vi "Calculate Derived Data.vi"(8 "error in":errorcluster, 11 "CVT":map{string, string}(c390)) -> (0 "error out":errorcluster, 3 "CVT Out":map{string, dbl}(c390))   [LabVIEW 2025]
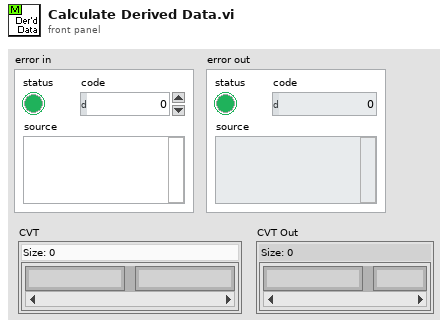
[diagram p1: front panel]
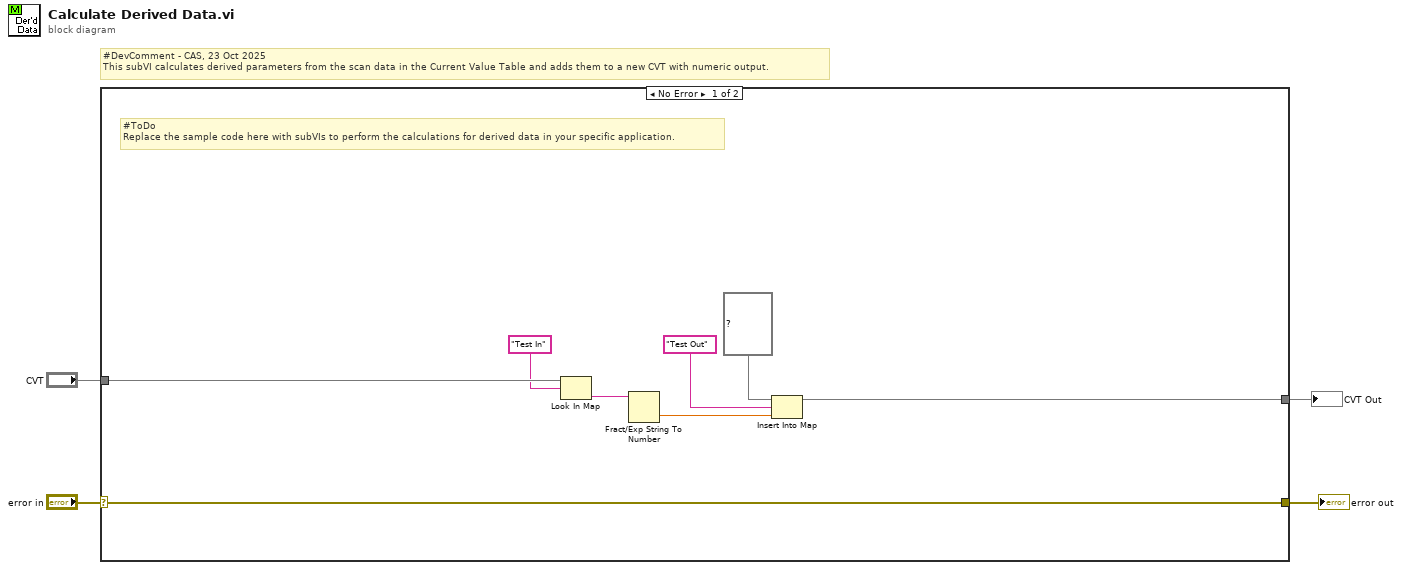
[diagram p0: block diagram]
diagram:
  # "#DevComment - CAS, 23 Oct 2025\nThis subVI calculates derived parameters from the scan data in the Current Value Table and adds them to a new CVT with numeric output."
  n1 = case shown="No Error" "error in" {
    selector: "error in" -> [w12 w13]
    tunnel: [w12 w13] -> w3
    tunnel: "CVT" -> [w11 _]
    tunnel: [w5 _] -> w1
    frame No Error {
      # "#ToDo\nReplace the sample code here with subVIs to perform the calculations for derived data in your specific application."
      n2 = Look In Map(map=w11, key="Test In") -> (value=w10:string)  [unwired: 1 in, 1 out]
      n3 = Fract/Exp String To Number(string=w10) -> (number=w9:dbl)  [unwired: 3 in, 1 out]
      n4 = Insert Into Map(map in=map{string, dbl} {} ("CVT Out"), key="Test Out", value=w9) -> (map out=w5:map{string, dbl})  [unwired: 2 out]
    }
    frame Error {
    }
  }
  "error out" <- w3
  "CVT Out" <- w1
